vi "Bitmap_File_Writer.vi"   [LabVIEW 2013]
types:
  T1 = enum16{"open", "replace", "create", "open or create", "replace or create", "replace or create with confirmation"}
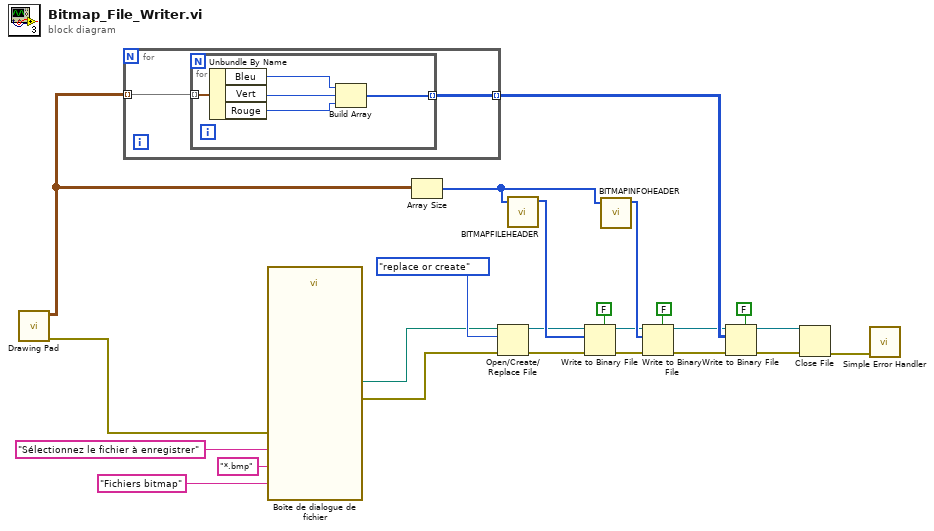
[diagram p0: block diagram]
diagram:
  n1 = call "Drawing Pad.vi"() -> ("sortie d'erreur"=w18:errorcluster, "Données image"=w8:cluster{"Rouge":u8, "Vert":u8, "Bleu":u8}[][])  [unwired: 10 in]
  n2 = for {
    tunnel: w8 -> [w26] mode=indexing
    tunnel: [w25] -> w6 mode=indexing
    n3 = for {
      tunnel: w26 -> [w28] mode=indexing
      tunnel: [w27] -> w25 mode=indexing
      n4 = Unbundle By Name(w28) -> ("Bleu"=w31:u8, "Vert"=w30:u8, "Rouge"=w29:u8)
      n5 = Build Array(w31, w30, w29) -> (w27:u8[])
    }
  }
  n6 = call "Boîte de dialogue de fichier"("prompt"="Sélectionnez le fichier à enregistrer", "error in"=w18, "pattern (all files)"="*.bmp", "pattern label"="Fichiers bitmap") -> ("selected path"=w20:path, "error out"=w19:errorcluster)  [unwired: 8 in, 2 out]
  n7 = Array Size(array=w8) -> (size(s)=w13:i32[])
  n8 = Open/Create/Replace File(file path (use dialog)=w20, error in=w19, operation (0:open)=T1."replace or create" ("opération (0 : open)")) -> (refnum out=w10:refnum<file>, error out=w15:errorcluster)  [unwired: 3 in, 1 out]
  n9 = call "BITMAPFILEHEADER.vi"("Dimensions de l'image"=w13) -> ("EN-TÊTE_FICHIER_BITMAP"=w12:u8[])  [unwired: 10 in]
  n10 = Write to Binary File(file (use dialog)=w10, data=w12, error in=w15, 5:FALSE ("ajouter une taille de tableau ou de chaîne ? (V)")) -> (refnum out=w9:refnum<file>, error out=w14:errorcluster)  [unwired: 2 in, 1 out]
  n11 = call "BITMAPINFOHEADER.vi"("Dimensions de l'image"=w13) -> ("EN-TÊTE_FICHIER_BITMAP"=w11:u8[])  [unwired: 10 in]
  n12 = Write to Binary File(file (use dialog)=w9, data=w11, error in=w14, 5:FALSE ("ajouter une taille de tableau ou de chaîne ? (V)")) -> (refnum out=w5:refnum<file>, error out=w4:errorcluster)  [unwired: 2 in, 1 out]
  n13 = Write to Binary File(file (use dialog)=w5, data=w6, error in=w4, 5:FALSE ("ajouter une taille de tableau ou de chaîne ? (V)")) -> (refnum out=w3:refnum<file>, error out=w2:errorcluster)  [unwired: 2 in, 1 out]
  n14 = Close File(refnum=w3, error in=w2) -> (error out=w1:errorcluster)  [unwired: 1 out]
  n15 = call <vilib>:"Simple Error Handler.vi"("error in (no error)"=w1) -> ()  [unwired: 4 in, 5 out]
